vi "ATF-Edit Channel Name list.vi"() -> ()   [LabVIEW 2022 SP3]
uses:
  Controls/SeCrTs-Edit CHN names.ctl
panel:
  out "Signal names":string[][](array[string])
  in  "Exit":bool
  in  "Save":bool
  in  "Select file to Edit":path
  out "List":string[](array[string])
  in  "Listbox":i32(listbox)
  in  "Tab Control":enum32{"Add New Name", "Rename"}(tab)
  in  "Add to list":bool
  in  "Channel Name":string[](array[string])
  in  "Enter New Name":string
  in  "Choose Channel names":string(combo)
  in  "Rename":bool
  in  "Delete":bool
  # "Channel Name Editor"
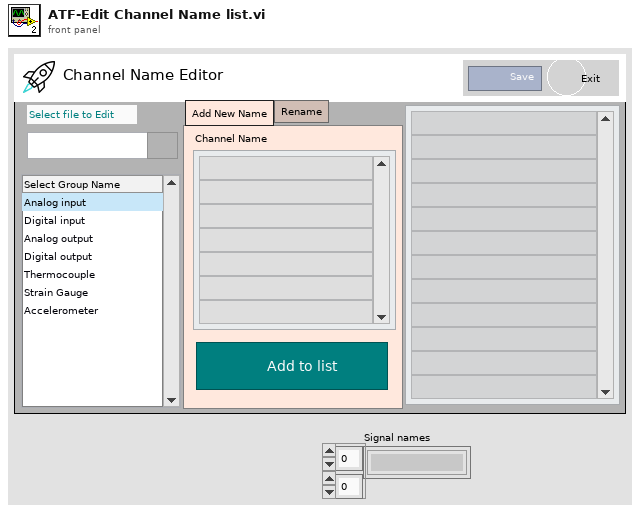
[diagram p1: front panel]
types:
  T1 = typedef "SeCrTs-Edit CHN names.ctl" = enum16{"initialize", "select group", "rename", "add to list", "pollevent", "Quit", "Save", "Read"}
  T2 = cluster{"path":path, "Data":string[][], "Group":i32}
  T3 = enum16{"open", "replace", "create", "open or create", "replace or create", "replace or create with confirmation"}
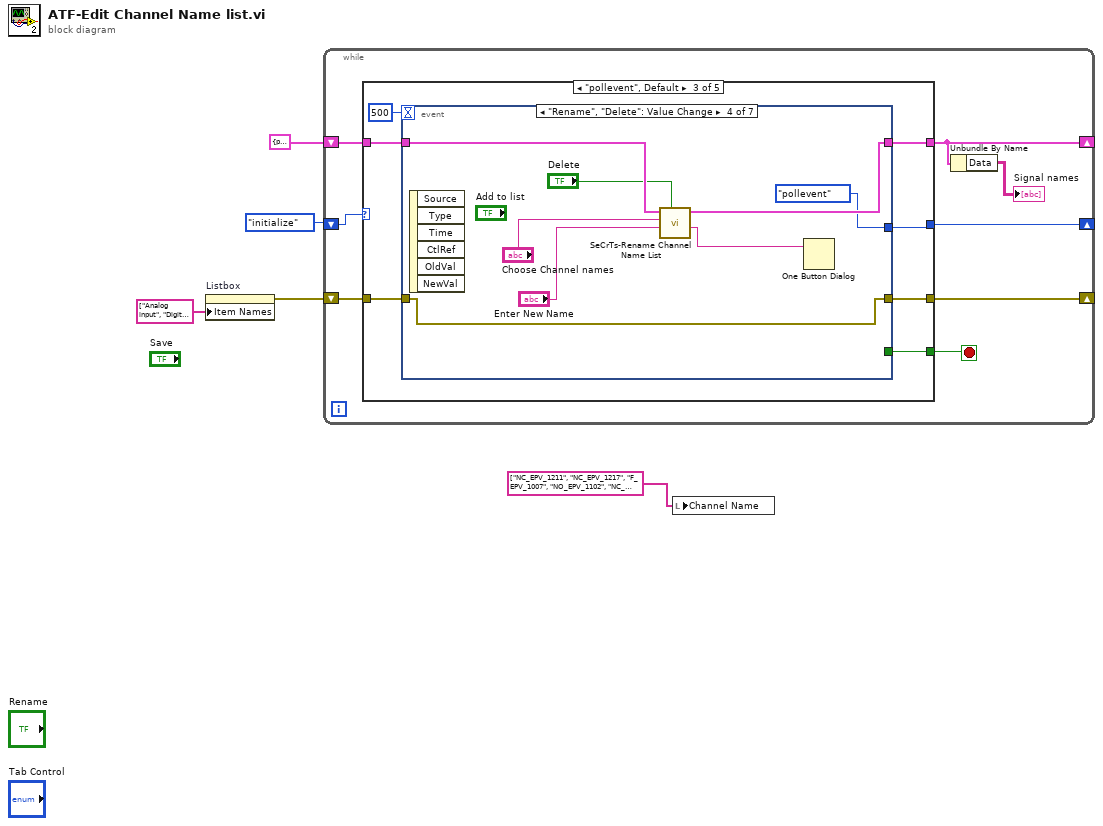
[diagram p0: block diagram]
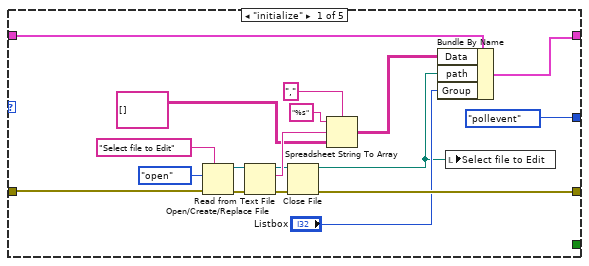
[diagram p2: hidden frame]
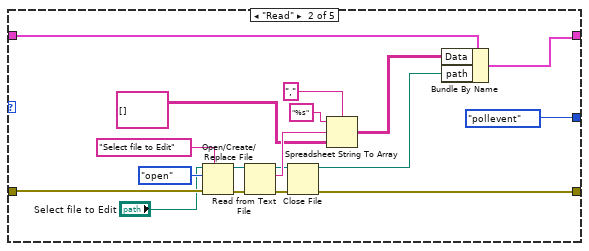
[diagram p3: hidden frame]
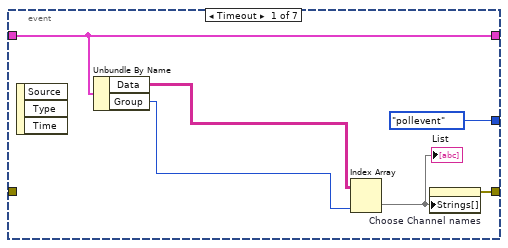
[diagram p4: hidden frame]
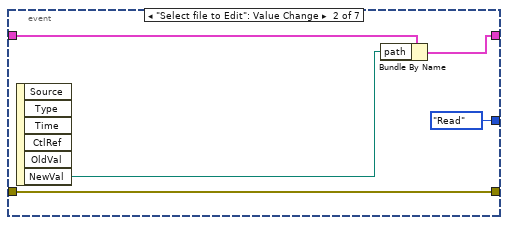
[diagram p5: hidden frame]
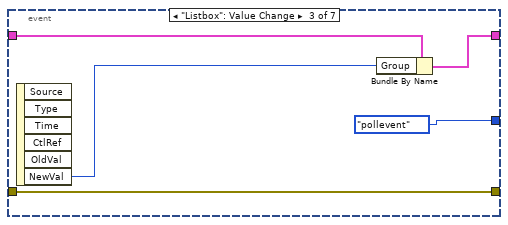
[diagram p6: hidden frame]
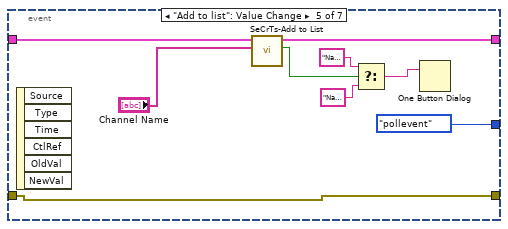
[diagram p7: hidden frame]
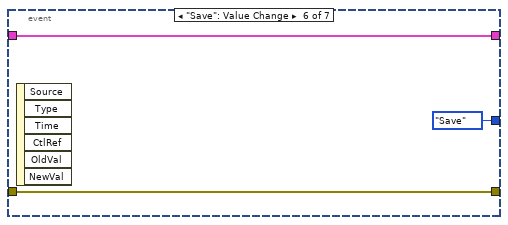
[diagram p8: hidden frame]
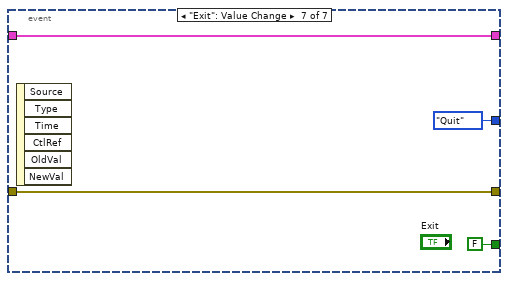
[diagram p9: hidden frame]
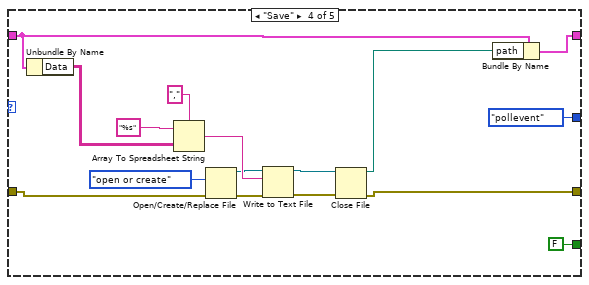
[diagram p10: hidden frame]
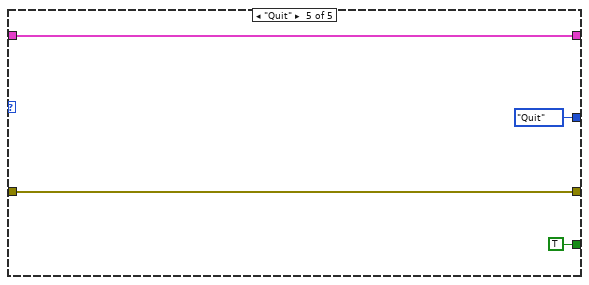
[diagram p11: hidden frame]
diagram:
  n1 = property on="Listbox" class="LstBox (strict)"("Item Names"=string[] ["Analog input", "Digital input", "Analog output", "Digital output", "Thermocouple", "Strain Gauge", "Accelerometer"]) -> (error out=w4:errorcluster)  [unwired: 2 in, 1 out]
  n2 = while {
    shift-right: [w7] -> _
    shift-left: T2 {"path"=path "", "Data"=[], "Group"=0} -> [w12]
    shift-right: [w10] -> _
    shift-left: w4 -> [w11]
    shift-right: [w9] -> _
    shift-left: SeCrTs-Edit_CHN_names."initialize" -> [w13]
    stop <- w8 stop-if-true
    n3 = case shown="\"pollevent\", Default" w13 {
      tunnel: w12 -> [w19 w37 w56 w101 w113]
      tunnel: [w17 w35 w55 w104 w113] -> w7
      tunnel: w11 -> [w21 w39 w52 w105 w114]
      tunnel: [w20 w38 w53 w106 w114] -> w10
      tunnel: [SeCrTs-Edit_CHN_names."pollevent" SeCrTs-Edit_CHN_names."pollevent" w54 SeCrTs-Edit_CHN_names."pollevent" SeCrTs-Edit_CHN_names."Quit"] -> w9
      tunnel: [_ _ w50 FALSE ("Quit") TRUE ("Quit")] -> w8
      frame "initialize" {
        n4 = Open/Create/Replace File(error in=w21, prompt="Select file to Edit", operation (0:open)=T3."open") -> (refnum out=w28:refnum<file>, error out=w27:errorcluster)  [unwired: 3 in, 1 out]
        n5 = Read from Text File(file (use dialog)=w28, error in=w27) -> (refnum out=w30:refnum<file>, text=w31:string, error out=w29:errorcluster)  [unwired: 2 in, 1 out]
        n6 = Close File(refnum=w30, error in=w29) -> (path=w14:path, error out=w20:errorcluster)
        n7 = Spreadsheet String To Array(delimiter (Tab)=",", format string="%s", spreadsheet string=w31, array type (2D Dbl)=string[][] [] ("Table Control")) -> (array=w18:string[][])
        n8 = Bundle By Name(cluster=w19, "Data"=w18, "path"=w14, "Group"="Listbox") -> (w17:T2)
        n9 = local write "Select file to Edit"(w14) -> ()
      }
      frame "Read" {
        n10 = Open/Create/Replace File(file path (use dialog)="Select file to Edit", error in=w39, prompt="Select file to Edit", operation (0:open)=T3."open") -> (refnum out=w46:refnum<file>, error out=w45:errorcluster)  [unwired: 2 in, 1 out]
        n11 = Read from Text File(file (use dialog)=w46, error in=w45) -> (refnum out=w48:refnum<file>, text=w49:string, error out=w47:errorcluster)  [unwired: 2 in, 1 out]
        n12 = Close File(refnum=w48, error in=w47) -> (path=w34:path, error out=w38:errorcluster)
        n13 = Spreadsheet String To Array(delimiter (Tab)=",", format string="%s", spreadsheet string=w49, array type (2D Dbl)=string[][] [] ("Table Control")) -> (array=w36:string[][])
        n14 = Bundle By Name(cluster=w37, "Data"=w36, "path"=w34) -> (w35:T2)
      }
      frame "pollevent", Default {
        n15 = event shown="[3] \"Rename\", \"Delete\": Value Change" {
          selector: _ -> [_ _ _ _ _ _ _]
          dyn-events: _ -> [_ _ _ _ _ _ _]
          timeout: 500 -> [_ _ _ _ _ _ _]
          tunnel: w56 -> [w61 w66 w71 w79 w88 w92 w95]
          tunnel: [w61 w67 w72 w80 w89 w92 w95] -> w55
          tunnel: [SeCrTs-Edit_CHN_names."pollevent" SeCrTs-Edit_CHN_names."Read" SeCrTs-Edit_CHN_names."pollevent" SeCrTs-Edit_CHN_names."pollevent" SeCrTs-Edit_CHN_names."pollevent" SeCrTs-Edit_CHN_names."Save" SeCrTs-Edit_CHN_names."Quit"] -> w54
          tunnel: [w62 w63 w69 w76 w82 w90 w93] -> w53
          tunnel: w52 -> [_ w63 w69 w76 w82 w90 w93]
          tunnel: [_ _ _ _ _ _ FALSE ("Quit")] -> w50
          event Timeout {
            n16 = event-data() -> ()  [unwired: 1 in, 3 out]
            n17 = Unbundle By Name(w61) -> ("Data"=w60:string[][], "Group"=w58:i32)
            n18 = Index Array(array=w60, index (col)=w58) -> (element=w59:string[])  [unwired: 1 in]
            "List" <- w59
            n19 = property on="Choose Channel names" class="CmbBox"("Strings[]"=w59) -> (error out=w62:errorcluster)  [unwired: 2 in, 1 out]
          }
          event "Select file to Edit": Value Change {
            n20 = event-data() -> ("NewVal"=w65:path)  [unwired: 1 in, 5 out]
            n21 = Bundle By Name(cluster=w66, "path"=w65) -> (w67:T2)
          }
          event "Listbox": Value Change {
            n22 = event-data() -> ("NewVal"=w70:i32)  [unwired: 1 in, 5 out]
            n23 = Bundle By Name(cluster=w71, "Group"=w70) -> (w72:T2)
          }
          event "Rename", "Delete": Value Change {
            n24 = event-data() -> ()  [unwired: 1 in, 6 out]
            n25 = call "SeCrTs-Rename Channel Name List.vi"("delete (T)"="Delete", "Enter New Name"="Enter New Name", "Choose Channel names"="Choose Channel names", "Cluster in"=w79) -> ("dialog"=w73:string, "Cluster out"=w80:T2)  [unwired: 6 in]
            n26 = One Button Dialog(message=w73) -> ()  [unwired: 1 in, 1 out]
          }
          event "Add to list": Value Change {
            n27 = event-data() -> ()  [unwired: 1 in, 6 out]
            n28 = call "SeCrTs-Add to List.vi"("Enter Channel Name"="Channel Name", "Cluster in"=w88) -> ("Boolean"=w84:bool, "Cluster out"=w89:T2)  [unwired: 8 in]
            n29 = Select(t="Name You Entered is already Exist!" ("message"), s=w84, f="Name Successfully Changed.") -> (s? t:f=w86:string)
            n30 = One Button Dialog(message=w86) -> ()  [unwired: 1 in, 1 out]
          }
          event "Save": Value Change {
            n31 = event-data() -> ()  [unwired: 1 in, 6 out]
          }
          event "Exit": Value Change {
            n32 = event-data() -> ()  [unwired: 1 in, 6 out]
          }
        }
      }
      frame "Save" {
        n33 = Unbundle By Name(w101) -> ("Data"=w97:string[][])
        n34 = Array To Spreadsheet String(delimiter (Tab)=",", array=w97, 3:"%s" ("format string")) -> (spreadsheet string=w112:string)
        n35 = Open/Create/Replace File(error in=w105, operation (0:open)=T3."open or create") -> (refnum out=w111:refnum<file>, error out=w100:errorcluster)  [unwired: 4 in, 1 out]
        n36 = Write to Text File(file (use dialog)=w111, text=w112, error in=w100) -> (refnum out=w110:refnum<file>, error out=w99:errorcluster)  [unwired: 1 in, 1 out]
        n37 = Close File(refnum=w110, error in=w99) -> (path=w102:path, error out=w106:errorcluster)
        n38 = Bundle By Name(cluster=w101, "path"=w102) -> (w104:T2)
      }
      frame "Quit" {
      }
    }
    n39 = Unbundle By Name(w7) -> ("Data"=→"Signal names":string[][])
  }
  n40 = local write "Channel Name"(string[] ["NC_EPV_1211", "NC_EPV_1217", "F_EPV_1007", "NO_EPV_1102", "NC_EPV_1214", "NC_EPV_1207", "AC_Switch", "NC_EPV_481", "NO_EPV_478R", "NO_EPV_477", "NC_EPV_56", "NO_EPV_122", "NC_EPV_61", "NC_EPV_1001", "F_EPV_1004", "F_EPV_1008", "N_EPV_1091"] ("Array")) -> ()
